vi "Read Channel Settings.vi"(8 "error in (no error)":errorcluster, 11 ".NET Refnum in":refnum<k24>) -> (0 "error out":errorcluster, 1 "DefaultValue":dbl, 2 "Array":string[][](array[string]), 3 ".NET Refnum out":refnum<k24>)   [LabVIEW 2023, in "Waveform Analog Output System Explorer.lvlib"]
uses:
  Waveform Analog Output System Explorer.lvlib
  NationalInstruments.VeriStand.SystemDefinitionAPI
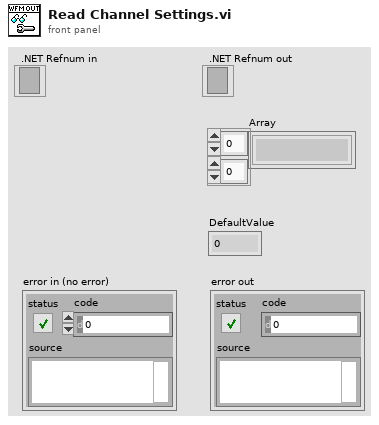
[diagram p1: front panel]
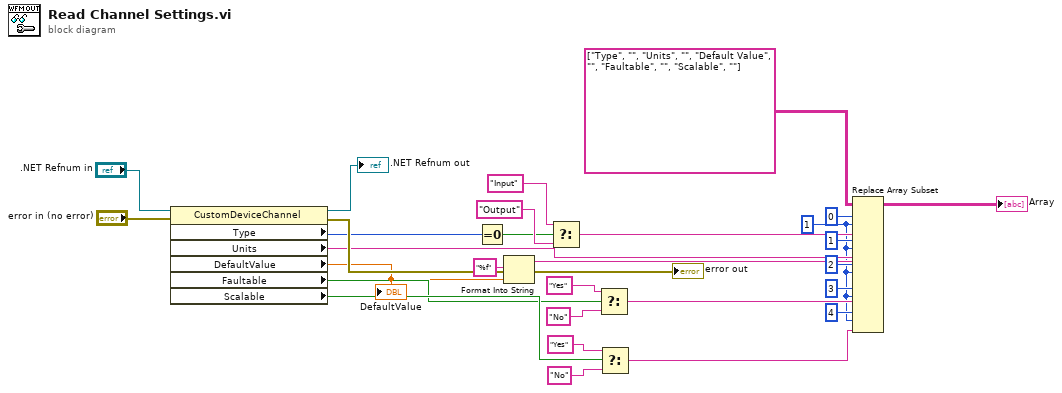
[diagram p0: block diagram]
diagram:
  w5 = 1 ("disabled index (col)")
  n1 = property class="CustomDeviceChannel"(reference=".NET Refnum in", error in="error in (no error)") -> (reference out=→".NET Refnum out":refnum<k24>, error out=w29:errorcluster, "Type"=w10:i32, "Units"=w15:string, "DefaultValue"=w16:dbl, "Faultable"=w19:bool, "Scalable"=w24:bool)
  "DefaultValue" <- w16
  n2 = Equal To 0?(x=w10) -> (x = 0?=w11:bool)
  n3 = Format Into String(format string="%f", error in=w29, w16) -> (resulting string=w18:string, error out=→"error out":errorcluster)  [unwired: 1 in]
  n4 = Select(t="Input", s=w11, f="Output") -> (s? t:f=w14:string)
  n5 = Select(t="Yes", s=w19, f="No") -> (s? t:f=w25:string)
  n6 = Select(t="Yes", s=w24, f="No") -> (s? t:f=w26:string)
  n7 = Replace Array Subset(array=string[][] [["Type", ""], ["Units", ""], ["Default Value", ""], ["Faultable", ""], ["Scalable", ""]], new element #1=w14, index (row) #1=0 ("index (row)"), index (col) #1=w5, new element #2=w15, index (row) #2=1 ("disabled index (row)"), index (col) #2=w5, new element #3=w18, index (row) #3=2 ("disabled index (row)"), index (col) #3=w5, new element #4=w25, index (row) #4=3 ("disabled index (row)"), index (col) #4=w5, new element #5=w26, index (row) #5=4 ("disabled index (row)"), index (col) #5=w5) -> (→"Array":string[][])
